vi "CloseDevice.vi"(2 "error in (no error)":errorcluster, 3 "nInputHandle":u64) -> (0 "error out":errorcluster, 1 "GX_STATUS":i32)   [LabVIEW 2016, in "GxLVLib.lvlib"]
uses:
  GxLVLib.lvlib
  GxIAPI.dll
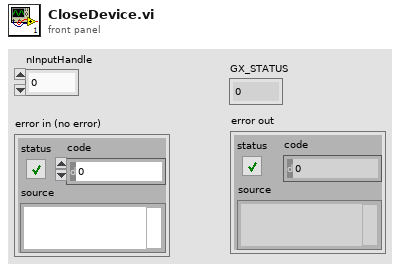
[diagram p1: front panel]
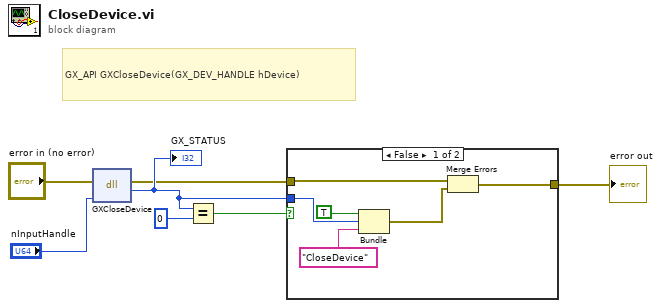
[diagram p0: block diagram]
diagram:
  # "GX_API GXCloseDevice(GX_DEV_HANDLE hDevice)"
  n1 = dll-call lib="GxIAPI.dll" fn="GXCloseDevice"(error in="error in (no error)", "hDevice"="nInputHandle") -> (error out=w1:errorcluster, "GX_STATUS"=w2:i32)  [unwired: 3 in, 1 out]
  "GX_STATUS" <- w2
  n2 = Equal?(x=w2, y=0) -> (x = y?=w3:bool)
  n3 = case shown="False" w3 {
    tunnel: w1 -> [w13 w14]
    tunnel: [w12 w14] -> w5
    tunnel: w2 -> [w10 _]
    frame False {
      n4 = Bundle(TRUE, "GX_STATUS"=w10, "CloseDevice") -> (w11:cluster{bool, "GX_STATUS":i32, string})  [unwired: 1 in]
      n5 = Merge Errors(w13, w11) -> (w12:errorcluster)
    }
    frame True {
    }
  }
  "error out" <- w5
